vi "RefNumFormat.vi"(0 "RefNum Val":u64) -> (1 "RefNum format ok?":bool, 2 "RefNum String":string)   [LabVIEW 2016]
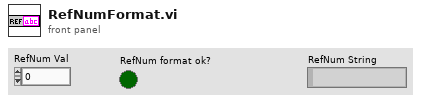
[diagram p1: front panel]
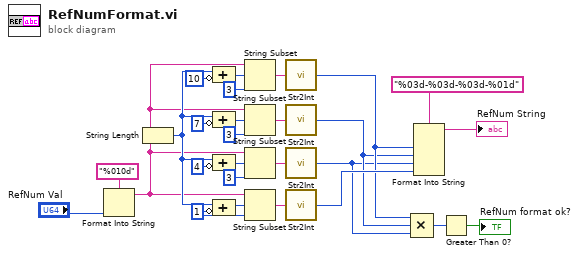
[diagram p0: block diagram]
diagram:
  w14 = 1 ("y")
  n1 = Format Into String(format string="%010d", "RefNum Val") -> (resulting string=w23:string)  [unwired: 2 in, 1 out]
  n2 = String Length(string=w23) -> (length=w24:i32)
  n3 = Compound Arithmetic op=ADD(w24, invert 10 ("y")) -> (w21:i32)
  n4 = Compound Arithmetic op=ADD(w24, invert 7 ("y")) -> (w16:i32)
  n5 = Compound Arithmetic op=ADD(w24, invert 4 ("y")) -> (w12:i32)
  n6 = Compound Arithmetic op=ADD(w24, invert w14) -> (w7:i32)
  n7 = String Subset(string=w23, offset (0)=w21, length (rest)=3 ("length (rest)")) -> (substring=w19:string)
  n8 = String Subset(string=w23, offset (0)=w16, length (rest)=3 ("length (rest)")) -> (substring=w18:string)
  n9 = String Subset(string=w23, offset (0)=w12, length (rest)=3 ("length (rest)")) -> (substring=w10:string)
  n10 = String Subset(string=w23, offset (0)=w7, length (rest)=w14) -> (substring=w8:string)
  n11 = call "Str2Int.vi"("string"=w19) -> ("Numeric"=w5:i32)
  n12 = call "Str2Int.vi"("string"=w18) -> ("Numeric"=w4:i32)
  n13 = call "Str2Int.vi"("string"=w10) -> ("Numeric"=w3:i32)
  n14 = call "Str2Int.vi"("string"=w8) -> ("Numeric"=w25:i32)
  n15 = Compound Arithmetic op=MULTIPLY(w5, w4, w3) -> (w2:i32)
  n16 = Format Into String(format string="%03d-%03d-%03d-%01d", w5, w4, w3, w25) -> (resulting string=→"RefNum String":string)  [unwired: 2 in, 1 out]
  n17 = Greater Than 0?(x=w2) -> (x > 0?=→"RefNum format ok?":bool)
